vi "2SMPP-02 Calibration.vi"(2 "error in (no error)":errorcluster, 3 "Sensor Voltage":dbl) -> (0 "error out":errorcluster, 1 "Pressure":dbl)   [LabVIEW 2017]
uses:
  <vilib>/gmath/NI_Gmath.lvlib
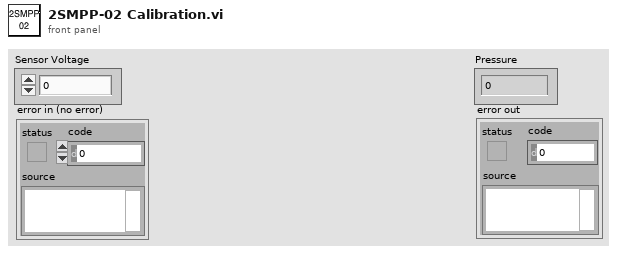
[diagram p1: front panel]
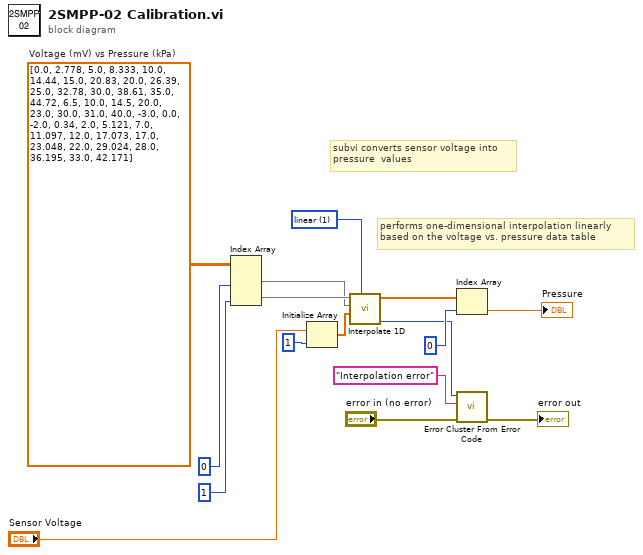
[diagram p0: block diagram]
diagram:
  w8 = 1 items=["nearest", "linear", "spline", "cubic Hermite", "Lagrange"] ("method")
  w16 = dbl[][] [[0.0, 2.778], [5.0, 8.333], [10.0, 14.44], [15.0, 20.83], [20.0, 26.39], [25.0, 32.78], [30.0, 38.61], [35.0, 44.72], [6.5, 10.0], [14.5, 20.0], [23.0, 30.0], [31.0, 40.0], [-3.0, 0.0], [-2.0, 0.34], [2.0, 5.121], [7.0, 11.097], [12.0, 17.073], [17.0, 23.048], [22.0, 29.024], [28.0, 36.195], [33.0, 42.171]]  # Voltage (mV) vs Pressure (kPa)
  # "performs one-dimensional interpolation linearly\nbased on the voltage vs. pressure data table"
  # "subvi converts sensor voltage into \npressure  values"
  n1 = Index Array "Index Array"(array=w16, index (col) #1=0 ("disabled index (col)"), index (col) #2=1 ("index (col)")) -> (element #1=w12:dbl[], element #2=w13:dbl[])  [unwired: 2 in]
  n2 = Initialize Array "Initialize Array"("Sensor Voltage", 1 ("dimension size")) -> (w10:dbl[])
  n3 = call <vilib>:"Interpolate 1D.vi"("method"=w8, "xi"=w10, "X"=w12, "Y"=w13) -> ("error"=w4:i32, "yi"=w7:dbl[])  [unwired: 5 in, 1 out]
  n4 = Index Array "Index Array"(array=w7, index=0) -> (element=→"Pressure":dbl)
  n5 = call <vilib>:"Error Cluster From Error Code.vi"("error in (no error)"="error in (no error)", "error message (\"\")"="Interpolation error" ("error message (\"\")"), "error code (0)"=w4) -> ("error out"=→"error out":errorcluster)  [unwired: 6 in]
